vi "MaxCharge.vi"() -> (2 "Max SOC":sgl)   [LabVIEW 2014]
panel:
  out "hour":u16
  out "Minute":u16
  out "month":u16
  out "day":u16
  out "year":u16
  out "Time, minutes":i32
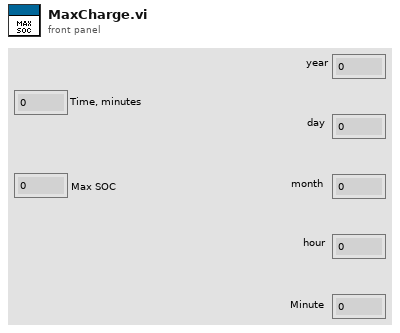
[diagram p1: front panel]
types:
  T1 = typedef "LVDateTimeRec.ctl" = cluster{"fractional second":dbl, "second":i32, "minute":i32, "hour":i32, "day of month":i32, "month":i32, "year":i32, "day of week":i32, "day of year":i32, "DST":i32}
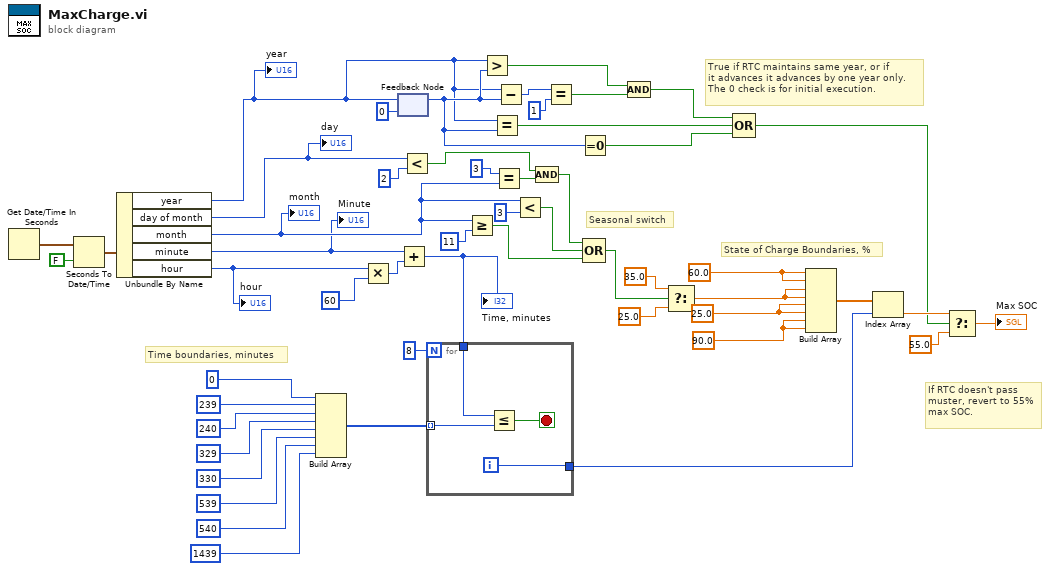
[diagram p0: block diagram]
diagram:
  w33 = sgl 90.0 ("element")
  w1 = sgl 25.0 ("element")
  w42 = sgl 60.0 ("element")
  # "Seasonal switch"
  # "True if RTC maintains same year, or if\nit advances it advances by one year only.\nThe 0 check is for initial execution."
  # "If RTC doesn't pass\nmuster, revert to 55%\nmax SOC."
  # "State of Charge Boundaries, %"
  # "Time boundaries, minutes"
  n1 = Get Date/Time In Seconds() -> (seconds since 1Jan1904=w52:timestamp)
  n2 = Seconds To Date/Time(time stamp (now)=w52, to UTC (F)=FALSE) -> (date time rec=w50:T1)
  n3 = Unbundle By Name(w50) -> ("year"=w7:i32, "day of month"=w6:i32, "month"=w5:i32, "minute"=w3:i32, "hour"=w4:i32)
  "year" <- w7
  "day" <- w6
  "month" <- w5
  "Minute" <- w3
  "hour" <- w4
  n4 = Build Array(0 ("element"), 239 ("element"), 240 ("element"), 329 ("element"), 330 ("element"), 539 ("element"), 540 ("element"), 1439 ("element")) -> (w49:i32[])
  n5 = Multiply(x=w4, y=60) -> (x*y=w47:i32)
  n6 = feedback-in #1(w7) -> ()
  n7 = feedback #1(0 ("year")) -> (w14:i32)
  n8 = Add(x=w3, y=w47) -> (x+y=w46:i32)
  "Time, minutes" <- w46
  n9 = Less?(x=w6, y=2) -> (x < y?=w25:bool)
  n10 = for {
    N: 8 -> [_]
    tunnel: w49 -> [w55] mode=indexing
    tunnel: w46 -> [w56]
    tunnel: [w53] -> w43
    i -> [w53]
    stop <- w54 stop-if-true
    n11 = Less Or Equal?(x=w56, y=w55) -> (x <= y?=w54:bool)
  }
  n12 = Greater Or Equal?(x=w5, y=11) -> (x >= y?=w29:bool)
  n13 = Greater?(x=w7, y=w14) -> (0:w18:bool)
  n14 = Equal?(x=w7, y=w14) -> (x = y?=w13:bool)
  n15 = Equal?(x=3, y=w5) -> (x = y?=w26:bool)
  n16 = Subtract(x=w7, y=w14) -> (x-y=w17:i32)
  n17 = Less?(x=w5, y=3) -> (x < y?=w23:bool)
  n18 = Compound Arithmetic op=AND(w25, w26) -> (w22:bool)
  n19 = Equal?(x=w17, y=1) -> (x = y?=w15:bool)
  n20 = Equal To 0?(x=w14) -> (x = 0?=w19:bool)
  n21 = Compound Arithmetic op=OR(w22, w23, w29) -> (w21:bool)
  n22 = Compound Arithmetic op=AND(w18, w15) -> (w12:bool)
  n23 = Select(t=sgl 35.0 ("element"), s=w21, f=sgl 25.0 ("element")) -> (s? t:f=w2:sgl)
  n24 = Compound Arithmetic op=OR(w12, w13, w19) -> (w8:bool)
  n25 = Build Array(w42, w42, w2, w2, w1, w1, w33, w33) -> (w44:sgl[])
  n26 = Index Array(array=w44, index=w43) -> (element=w11:sgl)
  n27 = Select(t=w11, s=w8, f=sgl 55.0) -> (s? t:f=→"Max SOC":sgl)
